vi "SendNotification.vi"(8 "error in (no error)":errorcluster, 11 "VIActivation in":refnum<class "VIActivation.lvclass">) -> (0 "error out":errorcluster, 3 "VIActivation out":refnum<class "VIActivation.lvclass">)   [LabVIEW 2021]
uses:
  b8ce3df6-1d66-406f-b005-46e60a7b74d5.vi
  VIActivation.lvclass
  C:/Users/Dany/OneDrive/LabVIEW/Class/ClassUtilities/ClassByRef/ClassByRef.lvclass
  C:/Users/Dany/OneDrive/LabVIEW/Class/VIActivation/VIActivation.lvclass
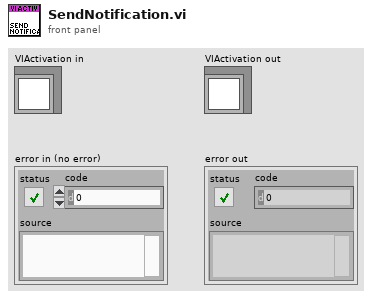
[diagram p1: front panel]
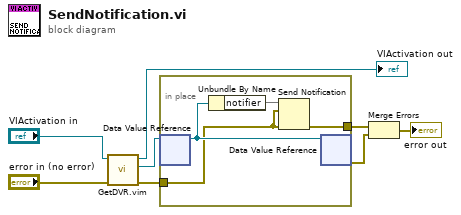
[diagram p0: block diagram]
diagram:
  n1 = call "GetDVR.vim"("error in (no error)"="error in (no error)", "ByRefClass in"="VIActivation in") -> ("error out"=w5:errorcluster, "DVR"=w7:refnum<data-value>, "ByRefClass out"=→"VIActivation out":refnum<class "VIActivation.lvclass">)  [unwired: 7 in]
  n2 = in-place {
    in-place-border: w5 -> [w9]
    in-place-border: [w11] -> w4
    n3 = in-place-dvr #1(w7) -> (w12:refnum<class "VIActivation.lvclass">)  [unwired: 1 out]
    n4 = Unbundle By Name(w12) -> ("notifier"=w10)
    n5 = Send Notification(notification=w9, notifier=w10, error in (no error)=w9) -> (error out=w11:errorcluster)  [unwired: 1 out]
    n6 = in-place-dvr #1(w12) -> (w3:errorcluster)  [unwired: 1 out]
  }
  n7 = Merge Errors(w4, w3) -> (→"error out":errorcluster)
